vi "vy_animated_generater.vi"(4 "new attribute":T1(ring)=enum."grey", 5 "chage_leave":i32=-1, 6 "leaves":T3={"names"=["Cube", "Pyramid", "Sphere"], "shapes"=[[{"xyzd"=[1.0, 1.0, 1.0, 1.0], "attribute"=enum."red", "prev. Ind."=[0, 0]}, {"xyzd"=[-1.0, 1.0, 1.0, 1.0], "attribute"=enum."red", "prev. Ind."=[0, 0]}, {"xyzd"=[1.0, -1.0, 1.0, 1.0], "attribute"=enum."pink", "prev. Ind."=[-1, -2]}, {"xyzd"=[-1.0, -1.0, 1.0, 1.0], "attribute"=enum."pink", "prev. Ind."=[-2, -1]}, {"xyzd"=[-1.0, -1.0, -1.0, 1.0], "attribute"=enum."red", "prev. Ind."=[-3, -1]}, {"xyzd"=[-1.0, 1.0, -1.0, 1.0], "attribute"=enum."red", "prev. Ind."=[-4, -1]}, {"xyzd"=[1.0, -1.0, -1.0, 1.0], "attribute"=enum."red", "prev. Ind."=[-4, -6]}, {"xyzd"=[1.0, 1.0, -1.0, 1.0], "attribute"=enum."red", "prev. Ind."=[-1, -7]}, {"xyzd"=[-1.0, 1.0, -1.0, 1.0], "attribute"=enum."blue", "prev. Ind."=[-2, -1]}, {"xyzd"=[-1.0, -1.0, -1.0, 1.0], "attribute"=enum."blue", "prev. Ind."=[-3, -1]}, {"xyzd"=[1.0, -1.0, 1.0, 1.0], "attribute"=enum."yellow", "prev. Ind."=[-4, -6]}, {"xyzd"=[1.0, -1.0, 1.0, 1.0], "attribute"=enum."yellow", "prev. Ind."=[-2, -8]}, {"xyzd"=[1.0, 1.0, -1.0, 1.0], "attribute"=enum."green", "prev. Ind."=[-11, -4]}, {"xyzd"=[1.0, 1.0, -1.0, 1.0], "attribute"=enum."green", "prev. Ind."=[-13, -12]}, {"xyzd"=[], "attribute"=enum."none", "prev. Ind."=[]}, {"xyzd"=[], "attribute"=enum."none", "prev. Ind."=[]}, {"xyzd"=[], "attribute"=enum."none", "prev. Ind."=[]}, {"xyzd"=[], "attribute"=enum."none", "prev. Ind."=[]}, {"xyzd"=[], "attribute"=enum."none", "prev. Ind."=[]}, {"xyzd"=[], "attribute"=enum."none", "prev. Ind."=[]}, {"xyzd"=[], "attribute"=enum."none", "prev. Ind."=[]}, {"xyzd"=[], "attribute"=enum."none", "prev. Ind."=[]}, {"xyzd"=[], "attribute"=enum."none", "prev. Ind."=[]}, {"xyzd"=[], "attribute"=enum."none", "prev. Ind."=[]}, {"xyzd"=[], "attribute"=enum."none", "prev. Ind."=[]}, {"xyzd"=[], "attribute"=enum."none", "prev. Ind."=[]}, {"xyzd"=[], "attribute"=enum."none", "prev. Ind."=[]}, {"xyzd"=[], "attribute"=enum."none", "prev. Ind."=[]}, {"xyzd"=[], "attribute"=enum."none", "prev. Ind."=[]}, {"xyzd"=[], "attribute"=enum."none", "prev. Ind."=[]}, {"xyzd"=[], "attribute"=enum."none", "prev. Ind."=[]}, {"xyzd"=[], "attribute"=enum."none", "prev. Ind."=[]}, {"xyzd"=[], "attribute"=enum."none", "prev. Ind."=[]}, {"xyzd"=[], "attribute"=enum."none", "prev. Ind."=[]}, {"xyzd"=[], "attribute"=enum."none", "prev. Ind."=[]}, {"xyzd"=[], "attribute"=enum."none", "prev. Ind."=[]}, {"xyzd"=[], "attribute"=enum."none", "prev. Ind."=[]}, {"xyzd"=[], "attribute"=enum."none", "prev. Ind."=[]}, {"xyzd"=[], "attribute"=enum."none", "prev. Ind."=[]}, {"xyzd"=[], "attribute"=enum."none", "prev. Ind."=[]}, {"xyzd"=[], "attribute"=enum."none", "prev. Ind."=[]}, {"xyzd"=[], "attribute"=enum."none", "prev. Ind."=[]}, {"xyzd"=[], "attribute"=enum."none", "prev. Ind."=[]}, {"xyzd"=[], "attribute"=enum."none", "prev. Ind."=[]}, {"xyzd"=[], "attribute"=enum."none", "prev. Ind."=[]}, {"xyzd"=[], "attribute"=enum."none", "prev. Ind."=[]}, {"xyzd"=[], "attribute"=enum."none", "prev. Ind."=[]}, {"xyzd"=[], "attribute"=enum."none", "prev. Ind."=[]}, {"xyzd"=[], "attribute"=enum."none", "prev. Ind."=[]}, {"xyzd"=[], "attribute"=enum."none", "prev. Ind."=[]}, {"xyzd"=[], "attribute"=enum."none", "prev. Ind."=[]}, {"xyzd"=[], "attribute"=enum."none", "prev. Ind."=[]}, {"xyzd"=[], "attribute"=enum."none", "prev. Ind."=[]}, {"xyzd"=[], "attribute"=enum."none", "prev. Ind."=[]}, {"xyzd"=[], "attribute"=enum."none", "prev. Ind."=[]}, {"xyzd"=[], "attribute"=enum."none", "prev. Ind."=[]}, {"xyzd"=[], "attribute"=enum."none", "prev. Ind."=[]}, {"xyzd"=[], "attribute"=enum."none", "prev. Ind."=[]}, {"xyzd"=[], "attribute"=enum."none", "prev. Ind."=[]}, {"xyzd"=[], "attribute"=enum."none", "prev. Ind."=[]}, {"xyzd"=[], "attribute"=enum."none", "prev. Ind."=[]}, {"xyzd"=[], "attribute"=enum."none", "prev. Ind."=[]}, {"xyzd"=[], "attribute"=enum."none", "prev. Ind."=[]}, {"xyzd"=[], "attribute"=enum."none", "prev. Ind."=[]}, {"xyzd"=[], "attribute"=enum."none", "prev. Ind."=[]}, {"xyzd"=[], "attribute"=enum."none", "prev. Ind."=[]}, {"xyzd"=[], "attribute"=enum."none", "prev. Ind."=[]}, {"xyzd"=[], "attribute"=enum."none", "prev. Ind."=[]}, {"xyzd"=[], "attribute"=enum."none", "prev. Ind."=[]}, {"xyzd"=[], "attribute"=enum."none", "prev. Ind."=[]}, {"xyzd"=[], "attribute"=enum."none", "prev. Ind."=[]}, {"xyzd"=[], "attribute"=enum."none", "prev. Ind."=[]}, {"xyzd"=[], "attribute"=enum."none", "prev. Ind."=[]}, {"xyzd"=[], "attribute"=enum."none", "prev. Ind."=[]}, {"xyzd"=[], "attribute"=enum."none", "prev. Ind."=[]}, {"xyzd"=[], "attribute"=enum."none", "prev. Ind."=[]}, {"xyzd"=[], "attribute"=enum."none", "prev. Ind."=[]}, {"xyzd"=[], "attribute"=enum."none", "prev. Ind."=[]}, {"xyzd"=[], "attribute"=enum."none", "prev. Ind."=[]}, {"xyzd"=[], "attribute"=enum."none", "prev. Ind."=[]}], [{"xyzd"=[1.0, 1.0, 1.0, 1.0], "attribute"=enum."red", "prev. Ind."=[0, 0]}, {"xyzd"=[-1.0, 1.0, 1.0, 1.0], "attribute"=enum."red", "prev. Ind."=[0, 0]}, {"xyzd"=[1.0, -1.0, 1.0, 1.0], "attribute"=enum."red", "prev. Ind."=[-1, -2]}, {"xyzd"=[-1.0, -1.0, 1.0, 1.0], "attribute"=enum."red", "prev. Ind."=[-2, -1]}, {"xyzd"=[0.0, 0.0, -1.0, 1.0], "attribute"=enum."yellow", "prev. Ind."=[-4, -3]}, {"xyzd"=[0.0, 0.0, -1.0, 1.0], "attribute"=enum."red", "prev. Ind."=[-3, -5]}, {"xyzd"=[0.0, 0.0, -1.0, 1.0], "attribute"=enum."yellow", "prev. Ind."=[-3, -4]}, {"xyzd"=[0.0, 0.0, -1.0, 1.0], "attribute"=enum."red", "prev. Ind."=[-6, -4]}, {"xyzd"=[], "attribute"=enum."none", "prev. Ind."=[]}, {"xyzd"=[], "attribute"=enum."none", "prev. Ind."=[]}, {"xyzd"=[], "attribute"=enum."none", "prev. Ind."=[]}, {"xyzd"=[], "attribute"=enum."none", "prev. Ind."=[]}, {"xyzd"=[], "attribute"=enum."none", "prev. Ind."=[]}, {"xyzd"=[], "attribute"=enum."none", "prev. Ind."=[]}, {"xyzd"=[], "attribute"=enum."none", "prev. Ind."=[]}, {"xyzd"=[], "attribute"=enum."none", "prev. Ind."=[]}, {"xyzd"=[], "attribute"=enum."none", "prev. Ind."=[]}, {"xyzd"=[], "attribute"=enum."none", "prev. Ind."=[]}, {"xyzd"=[], "attribute"=enum."none", "prev. Ind."=[]}, {"xyzd"=[], "attribute"=enum."none", "prev. Ind."=[]}, {"xyzd"=[], "attribute"=enum."none", "prev. Ind."=[]}, {"xyzd"=[], "attribute"=enum."none", "prev. Ind."=[]}, {"xyzd"=[], "attribute"=enum."none", "prev. Ind."=[]}, {"xyzd"=[], "attribute"=enum."none", "prev. Ind."=[]}, {"xyzd"=[], "attribute"=enum."none", "prev. Ind."=[]}, {"xyzd"=[], "attribute"=enum."none", "prev. Ind."=[]}, {"xyzd"=[], "attribute"=enum."none", "prev. Ind."=[]}, {"xyzd"=[], "attribute"=enum."none", "prev. Ind."=[]}, {"xyzd"=[], "attribute"=enum."none", "prev. Ind."=[]}, {"xyzd"=[], "attribute"=enum."none", "prev. Ind."=[]}, {"xyzd"=[], "attribute"=enum."none", "prev. Ind."=[]}, {"xyzd"=[], "attribute"=enum."none", "prev. Ind."=[]}, {"xyzd"=[], "attribute"=enum."none", "prev. Ind."=[]}, {"xyzd"=[], "attribute"=enum."none", "prev. Ind."=[]}, {"xyzd"=[], "attribute"=enum."none", "prev. Ind."=[]}, {"xyzd"=[], "attribute"=enum."none", "prev. Ind."=[]}, {"xyzd"=[], "attribute"=enum."none", "prev. Ind."=[]}, {"xyzd"=[], "attribute"=enum."none", "prev. Ind."=[]}, {"xyzd"=[], "attribute"=enum."none", "prev. Ind."=[]}, {"xyzd"=[], "attribute"=enum."none", "prev. Ind."=[]}, {"xyzd"=[], "attribute"=enum."none", "prev. Ind."=[]}, {"xyzd"=[], "attribute"=enum."none", "prev. Ind."=[]}, {"xyzd"=[], "attribute"=enum."none", "prev. Ind."=[]}, {"xyzd"=[], "attribute"=enum."none", "prev. Ind."=[]}, {"xyzd"=[], "attribute"=enum."none", "prev. Ind."=[]}, {"xyzd"=[], "attribute"=enum."none", "prev. Ind."=[]}, {"xyzd"=[], "attribute"=enum."none", "prev. Ind."=[]}, {"xyzd"=[], "attribute"=enum."none", "prev. Ind."=[]}, {"xyzd"=[], "attribute"=enum."none", "prev. Ind."=[]}, {"xyzd"=[], "attribute"=enum."none", "prev. Ind."=[]}, {"xyzd"=[], "attribute"=enum."none", "prev. Ind."=[]}, {"xyzd"=[], "attribute"=enum."none", "prev. Ind."=[]}, {"xyzd"=[], "attribute"=enum."none", "prev. Ind."=[]}, {"xyzd"=[], "attribute"=enum."none", "prev. Ind."=[]}, {"xyzd"=[], "attribute"=enum."none", "prev. Ind."=[]}, {"xyzd"=[], "attribute"=enum."none", "prev. Ind."=[]}, {"xyzd"=[], "attribute"=enum."none", "prev. Ind."=[]}, {"xyzd"=[], "attribute"=enum."none", "prev. Ind."=[]}, {"xyzd"=[], "attribute"=enum."none", "prev. Ind."=[]}, {"xyzd"=[], "attribute"=enum."none", "prev. Ind."=[]}, {"xyzd"=[], "attribute"=enum."none", "prev. Ind."=[]}, {"xyzd"=[], "attribute"=enum."none", "prev. Ind."=[]}, {"xyzd"=[], "attribute"=enum."none", "prev. Ind."=[]}, {"xyzd"=[], "attribute"=enum."none", "prev. Ind."=[]}, {"xyzd"=[], "attribute"=enum."none", "prev. Ind."=[]}, {"xyzd"=[], "attribute"=enum."none", "prev. Ind."=[]}, {"xyzd"=[], "attribute"=enum."none", "prev. Ind."=[]}, {"xyzd"=[], "attribute"=enum."none", "prev. Ind."=[]}, {"xyzd"=[], "attribute"=enum."none", "prev. Ind."=[]}, {"xyzd"=[], "attribute"=enum."none", "prev. Ind."=[]}, {"xyzd"=[], "attribute"=enum."none", "prev. Ind."=[]}, {"xyzd"=[], "attribute"=enum."none", "prev. Ind."=[]}, {"xyzd"=[], "attribute"=enum."none", "prev. Ind."=[]}, {"xyzd"=[], "attribute"=enum."none", "prev. Ind."=[]}, {"xyzd"=[], "attribute"=enum."none", "prev. Ind."=[]}, {"xyzd"=[], "attribute"=enum."none", "prev. Ind."=[]}, {"xyzd"=[], "attribute"=enum."none", "prev. Ind."=[]}, {"xyzd"=[], "attribute"=enum."none", "prev. Ind."=[]}, {"xyzd"=[], "attribute"=enum."none", "prev. Ind."=[]}, {"xyzd"=[], "attribute"=enum."none", "prev. Ind."=[]}], [{"xyzd"=[-0.09090909090909091, 0.0, -1.0, 1.0], "attribute"=enum."red", "prev. Ind."=[0, 0]}, {"xyzd"=[0.09090909090909091, 0.0, -1.0, 1.0], "attribute"=enum."red", "prev. Ind."=[0, 0]}, {"xyzd"=[0.0, 0.09090909090909091, -1.0, 1.0], "attribute"=enum."red", "prev. Ind."=[-1, -2]}, {"xyzd"=[1.1132785034748885e-17, -0.09090909090909091, -1.0, 1.0], "attribute"=enum."red", "prev. Ind."=[-2, -3]}, {"xyzd"=[0.22076356771783573, 0.2162289295654466, -0.9510565162951535, 1.0], "attribute"=enum."red", "prev. Ind."=[-2, -3]}, {"xyzd"=[0.2162289295654466, -0.2207635677178357, -0.9510565162951535, 1.0], "attribute"=enum."red", "prev. Ind."=[-4, -2]}, {"xyzd"=[-0.2207635677178357, -0.21622892956544665, -0.9510565162951535, 1.0], "attribute"=enum."red", "prev. Ind."=[-3, -6]}, {"xyzd"=[-0.21622892956544673, 0.2207635677178356, -0.9510565162951535, 1.0], "attribute"=enum."red", "prev. Ind."=[-7, -5]}, {"xyzd"=[0.3494270285103859, 0.4726438982563176, -0.8090169943749475, 1.0], "attribute"=enum."red", "prev. Ind."=[-6, -4]}, {"xyzd"=[0.5873920684232319, 0.021495598758897283, -0.8090169943749475, 1.0], "attribute"=enum."red", "prev. Ind."=[-4, -5]}, {"xyzd"=[0.3830389001987991, -0.44583932503427814, -0.8090169943749475, 1.0], "attribute"=enum."red", "prev. Ind."=[-1, -5]}, {"xyzd"=[-0.10975037244495894, -0.5774481436118044, -0.8090169943749475, 1.0], "attribute"=enum."red", "prev. Ind."=[-6, -5]}, {"xyzd"=[-0.5198953761380584, -0.274226732254157, -0.8090169943749475, 1.0], "attribute"=enum."red", "prev. Ind."=[-1, -6]}, {"xyzd"=[-0.5385485576662208, 0.23549300169677978, -0.8090169943749475, 1.0], "attribute"=enum."red", "prev. Ind."=[-1, -6]}, {"xyzd"=[-0.1516636908831792, 0.5678817021882443, -0.8090169943749475, 1.0], "attribute"=enum."red", "prev. Ind."=[-1, -7]}, {"xyzd"=[0.6603788169001088, 0.467341754369419, -0.5877852522924731, 1.0], "attribute"=enum."red", "prev. Ind."=[-6, -7]}, {"xyzd"=[0.806281012237646, -0.06647876723067801, -0.5877852522924731, 1.0], "attribute"=enum."red", "prev. Ind."=[-1, -7]}, {"xyzd"=[0.5749153611338783, -0.5691931348143405, -0.5877852522924731, 1.0], "attribute"=enum."red", "prev. Ind."=[-1, -7]}, {"xyzd"=[0.07454042308304981, -0.805575708741316, -0.5877852522924731, 1.0], "attribute"=enum."red", "prev. Ind."=[-8, -7]}, {"xyzd"=[-0.46071280735286246, -0.6650204555714944, -0.5877852522924731, 1.0], "attribute"=enum."red", "prev. Ind."=[-7, -8]}, {"xyzd"=[-0.7803933949758588, -0.2132947403606729, -0.5877852522924731, 1.0], "attribute"=enum."red", "prev. Ind."=[-1, -8]}, {"xyzd"=[-0.7349192399831584, 0.33823395437189707, -0.5877852522924731, 1.0], "attribute"=enum."red", "prev. Ind."=[-1, -8]}, {"xyzd"=[-0.34556820488478407, 0.7314992228021719, -0.5877852522924731, 1.0], "attribute"=enum."red", "prev. Ind."=[-1, -8]}, {"xyzd"=[0.20547803384198088, 0.7824878751750135, -0.5877852522924731, 1.0], "attribute"=enum."red", "prev. Ind."=[-9, -15]}, {"xyzd"=[0.43703805980741456, 0.8446929805954613, -0.3090169943749474, 1.0], "attribute"=enum."red", "prev. Ind."=[-9, -1]}, {"xyzd"=[0.8243353153228079, 0.4743203401701433, -0.3090169943749474, 1.0], "attribute"=enum."red", "prev. Ind."=[-1, -10]}, {"xyzd"=[0.9499119326982213, -0.0466456568718201, -0.3090169943749474, 1.0], "attribute"=enum."red", "prev. Ind."=[-1, -10]}, {"xyzd"=[0.77389822319894, -0.5528019874394424, -0.3090169943749474, 1.0], "attribute"=enum."red", "prev. Ind."=[-1, -10]}, {"xyzd"=[0.3521772959375426, -0.8834475929072387, -0.3090169943749474, 1.0], "attribute"=enum."red", "prev. Ind."=[-11, -10]}, {"xyzd"=[-0.18135743441815916, -0.9336048297693927, -0.3090169943749474, 1.0], "attribute"=enum."red", "prev. Ind."=[-10, -11]}, {"xyzd"=[-0.657312460756494, -0.6873491297162718, -0.3090169943749474, 1.0], "attribute"=enum."red", "prev. Ind."=[-1, -11]}, {"xyzd"=[-0.9245754251525565, -0.22286493755510975, -0.3090169943749474, 1.0], "attribute"=enum."red", "prev. Ind."=[-1, -11]}, {"xyzd"=[-0.8982922248004648, 0.3123772975913979, -0.3090169943749474, 1.0], "attribute"=enum."red", "prev. Ind."=[-1, -11]}, {"xyzd"=[-0.5868075901037884, 0.7484419479051518, -0.3090169943749474, 1.0], "attribute"=enum."red", "prev. Ind."=[-12, -11]}, {"xyzd"=[-0.0890156917334638, 0.9468815679971211, -0.3090169943749474, 1.0], "attribute"=enum."red", "prev. Ind."=[-11, -12]}, {"xyzd"=[0.0, 1.0, 0.0, 1.0], "attribute"=enum."red", "prev. Ind."=[-11, -1]}, {"xyzd"=[0.49999999999999994, 0.8660254037844387, 0.0, 1.0], "attribute"=enum."red", "prev. Ind."=[-1, -12]}, {"xyzd"=[0.8660254037844386, 0.5000000000000001, 0.0, 1.0], "attribute"=enum."red", "prev. Ind."=[-1, -12]}, {"xyzd"=[1.0, 6.123031769111886e-17, 0.0, 1.0], "attribute"=enum."red", "prev. Ind."=[-1, -12]}, {"xyzd"=[0.8660254037844387, -0.4999999999999998, 0.0, 1.0], "attribute"=enum."red", "prev. Ind."=[-1, -12]}, {"xyzd"=[0.49999999999999994, -0.8660254037844387, 0.0, 1.0], "attribute"=enum."red", "prev. Ind."=[-1, -12]}, {"xyzd"=[1.2246063538223773e-16, -1.0, 0.0, 1.0], "attribute"=enum."red", "prev. Ind."=[-13, -12]}, {"xyzd"=[-0.5000000000000001, -0.8660254037844386, 0.0, 1.0], "attribute"=enum."red", "prev. Ind."=[-13, -12]}, {"xyzd"=[-0.8660254037844384, -0.5000000000000004, 0.0, 1.0], "attribute"=enum."red", "prev. Ind."=[-12, -13]}, {"xyzd"=[-1.0, -1.836909530733566e-16, 0.0, 1.0], "attribute"=enum."red", "prev. Ind."=[-12, -13]}, {"xyzd"=[-0.8660254037844386, 0.5000000000000001, 0.0, 1.0], "attribute"=enum."red", "prev. Ind."=[-12, -13]}, {"xyzd"=[-0.5000000000000004, 0.8660254037844384, 0.0, 1.0], "attribute"=enum."red", "prev. Ind."=[-1, -13]}, {"xyzd"=[0.0, 0.9510565162951535, 0.3090169943749474, 1.0], "attribute"=enum."red", "prev. Ind."=[-11, -12]}, {"xyzd"=[0.5141799724162847, 0.8000796542554137, 0.3090169943749474, 1.0], "attribute"=enum."red", "prev. Ind."=[-1, -12]}, {"xyzd"=[0.8651114366124775, 0.39508315508228004, 0.3090169943749474, 1.0], "attribute"=enum."red", "prev. Ind."=[-11, -12]}, {"xyzd"=[0.9413761322695258, -0.13534945430529863, 0.3090169943749474, 1.0], "attribute"=enum."red", "prev. Ind."=[-11, -12]}, {"xyzd"=[0.718760557376906, -0.6228095682844902, 0.3090169943749474, 1.0], "attribute"=enum."red", "prev. Ind."=[-11, -12]}, {"xyzd"=[0.2679435840365368, -0.9125320448954815, 0.3090169943749474, 1.0], "attribute"=enum."red", "prev. Ind."=[-11, -12]}, {"xyzd"=[-0.2679435840365362, -0.9125320448954817, 0.3090169943749474, 1.0], "attribute"=enum."red", "prev. Ind."=[-12, -11]}, {"xyzd"=[-0.7187605573769059, -0.6228095682844903, 0.3090169943749474, 1.0], "attribute"=enum."red", "prev. Ind."=[-12, -11]}, {"xyzd"=[-0.9413761322695257, -0.13534945430529882, 0.3090169943749474, 1.0], "attribute"=enum."red", "prev. Ind."=[-12, -11]}, {"xyzd"=[-0.8651114366124774, 0.39508315508228037, 0.3090169943749474, 1.0], "attribute"=enum."red", "prev. Ind."=[-12, -11]}, {"xyzd"=[-0.5141799724162853, 0.8000796542554134, 0.3090169943749474, 1.0], "attribute"=enum."red", "prev. Ind."=[-1, -11]}, {"xyzd"=[0.0, 0.8090169943749475, 0.5877852522924731, 1.0], "attribute"=enum."red", "prev. Ind."=[-10, -11]}, {"xyzd"=[0.5200261000100609, 0.619742972929746, 0.5877852522924731, 1.0], "attribute"=enum."red", "prev. Ind."=[-10, -11]}, {"xyzd"=[0.7967262083790821, 0.14048432677478692, 0.5877852522924731, 1.0], "attribute"=enum."none", "prev. Ind."=[-10, -11]}, {"xyzd"=[0.7006292692220368, -0.40450849718747356, 0.5877852522924731, 1.0], "attribute"=enum."none", "prev. Ind."=[-11, -10]}, {"xyzd"=[0.27670010836902137, -0.7602272997045328, 0.5877852522924731, 1.0], "attribute"=enum."none", "prev. Ind."=[-11, -10]}, {"xyzd"=[-0.2767001083690212, -0.760227299704533, 0.5877852522924731, 1.0], "attribute"=enum."none", "prev. Ind."=[-9, -10]}, {"xyzd"=[-0.7006292692220366, -0.40450849718747406, 0.5877852522924731, 1.0], "attribute"=enum."none", "prev. Ind."=[-9, -10]}, {"xyzd"=[-0.7967262083790823, 0.14048432677478656, 0.5877852522924731, 1.0], "attribute"=enum."red", "prev. Ind."=[-10, -9]}, {"xyzd"=[-0.5200261000100611, 0.6197429729297458, 0.5877852522924731, 1.0], "attribute"=enum."red", "prev. Ind."=[-10, -9]}, {"xyzd"=[0.0, 0.5877852522924731, 0.8090169943749475, 1.0], "attribute"=enum."red", "prev. Ind."=[-8, -9]}, {"xyzd"=[0.45954901517266916, 0.3664781104873198, 0.8090169943749475, 1.0], "attribute"=enum."red", "prev. Ind."=[-8, -9]}, {"xyzd"=[0.5730482488287673, -0.13079452330586896, 0.8090169943749475, 1.0], "attribute"=enum."red", "prev. Ind."=[-9, -8]}, {"xyzd"=[0.25503046306281557, -0.5295762133276872, 0.8090169943749475, 1.0], "attribute"=enum."red", "prev. Ind."=[-1, -8]}, {"xyzd"=[-0.2550304630628154, -0.5295762133276873, 0.8090169943749475, 1.0], "attribute"=enum."red", "prev. Ind."=[-1, -8]}, {"xyzd"=[-0.5730482488287673, -0.13079452330586913, 0.8090169943749475, 1.0], "attribute"=enum."red", "prev. Ind."=[-7, -8]}, {"xyzd"=[-0.4595490151726693, 0.3664781104873197, 0.8090169943749475, 1.0], "attribute"=enum."red", "prev. Ind."=[-8, -7]}, {"xyzd"=[0.0, 0.30901699437494745, 0.9510565162951535, 1.0], "attribute"=enum."red", "prev. Ind."=[-6, -7]}, {"xyzd"=[0.30901699437494745, 1.8921208737532724e-17, 0.9510565162951535, 1.0], "attribute"=enum."red", "prev. Ind."=[-7, -6]}, {"xyzd"=[3.784241747506545e-17, -0.30901699437494745, 0.9510565162951535, 1.0], "attribute"=enum."red", "prev. Ind."=[-5, -6]}, {"xyzd"=[-0.30901699437494745, -5.676362621259817e-17, 0.9510565162951535, 1.0], "attribute"=enum."red", "prev. Ind."=[-4, -5]}, {"xyzd"=[0.0, 0.09090909090909091, 1.0, 1.0], "attribute"=enum."red", "prev. Ind."=[-3, -4]}, {"xyzd"=[1.1132785034748885e-17, -0.09090909090909091, 1.0, 1.0], "attribute"=enum."red", "prev. Ind."=[-3, -1]}]]}, 7 "variables":dbl[](array[numeric])=[0.4925750394941765, 0.002174868167709741, 0.5074249605058234], 8 "vy_string":string="Structure  { s=(15,15,15)} [klossar {m=(,v1*3,) r=(30,v0*360,0)}  [Pyramid{r=(,,v0*360) m=(,,-4)} Cube {s=(1,v1,1) m=(,2-v1,)} Pyramid{r=(,180,v0*360) m=(,,4)}]  Cube{r=(45,v1*90,) m=(v1*5-2,-5,)}]", 9 "vy_in":T2(array[cluster])) -> (0 "selected leave":string, 3 "vy_out":T2(array[cluster]))   [LabVIEW 2011]
uses:
  <vilib>/Analysis/baseanly.llb/A x Vector.vi
  <vilib>/Analysis/NI_AALBase.lvlib
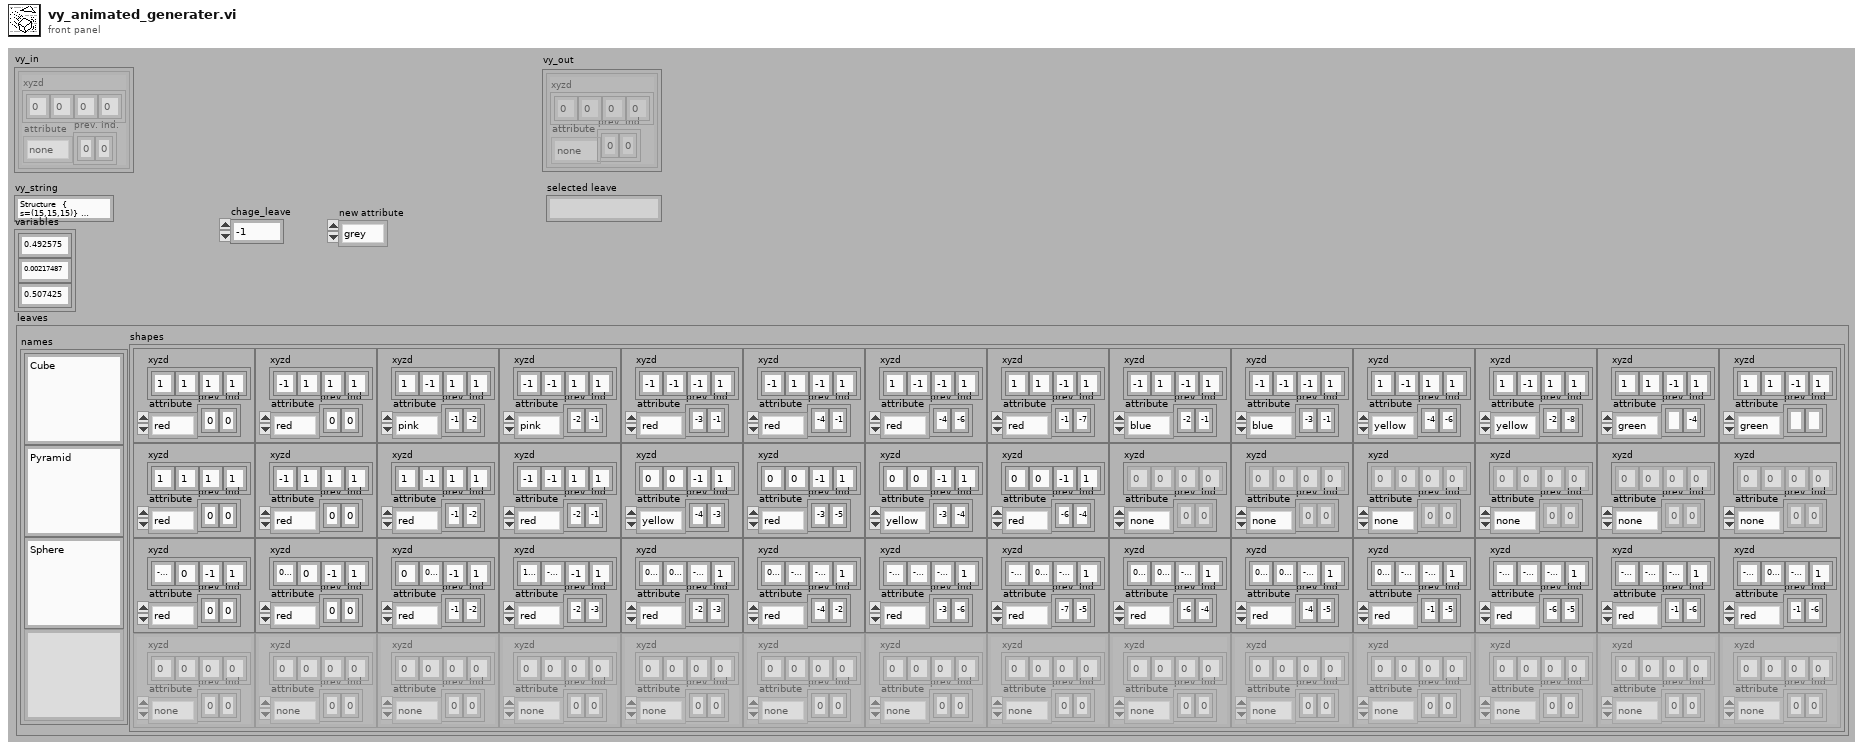
[diagram p1: front panel]
types:
  T1 = enum16{"none", "transparent", "reflective", "white", "black", "grey", "red", "yellow", "green", "blue", "pink"}
  T2 = cluster{"xyzd":dbl[], "attribute":enum16{"none", "transparent", "reflective", "white", "black", "grey", "red", "yellow", "green", "blue", "pink"}, "prev. Ind.":i16[]}[]
  T3 = cluster{"names":string[], "shapes":cluster{"xyzd":dbl[], "attribute":enum16{"none", "transparent", "reflective", "white", "black", "grey", "red", "yellow", "green", "blue", "pink"}, "prev. Ind.":i16[]}[][]}
  T4 = cluster{"xyzd":dbl[], "attribute":enum16{"none", "transparent", "reflective", "white", "black", "grey", "red", "yellow", "green", "blue", "pink"}, "prev. Ind.":i16[]}[][]
  T5 = cluster{"xyzd":dbl[], "attribute":enum16{"none", "transparent", "reflective", "white", "black", "grey", "red", "yellow", "green", "blue", "pink"}, "prev. Ind.":i16[]}
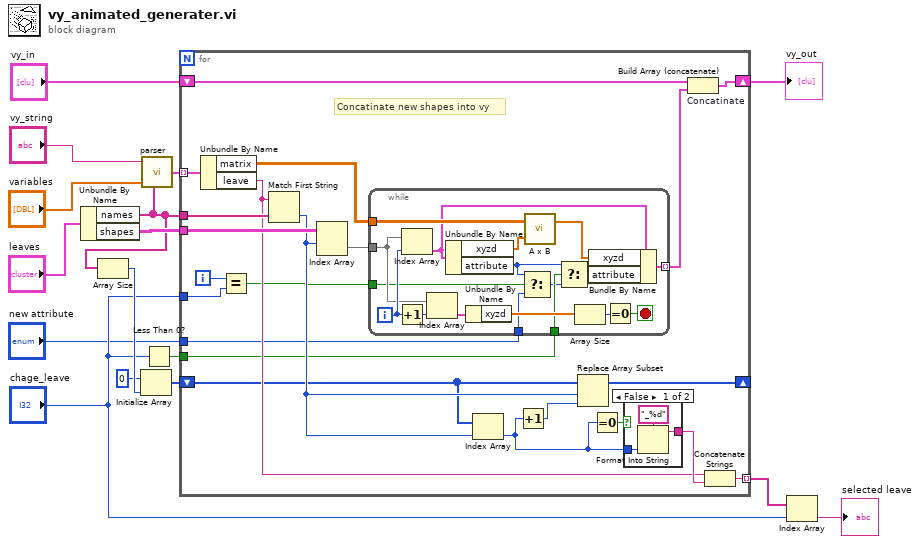
[diagram p0: block diagram]
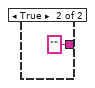
[diagram p2: hidden frame]
diagram:
  n1 = Unbundle By Name("leaves") -> ("names"=w12:string[], "shapes"=w14:T4)
  n2 = Array Size(array=w12) -> (size(s)=w11:i32)
  n3 = Initialize Array(0, w11) -> (w9:i32[])
  n4 = call "parser.vi"("in string"="vy_string", "variables"="variables", "leaves"=w12) -> ("leaves_projection_array"=w13:cluster{"matrix":dbl[][], "leave":string}[])  [unwired: 2 in]
  n5 = Less Than 0?(x="chage_leave") -> (x < 0?=w2:bool)
  n6 = for {
    tunnel: w13 -> [w38] mode=indexing
    tunnel: w12 -> [w37]
    tunnel: w14 -> [w36]
    shift-right: [w33] -> w6
    shift-left: "vy_in" -> [w32]
    tunnel: [w29] -> w5 mode=indexing
    shift-right: [w24] -> _
    shift-left: w9 -> [w25]
    tunnel: "chage_leave" -> [w20]
    tunnel: "new attribute" -> [w17]
    tunnel: w2 -> [w18]
    i -> [w21]
    # "Concatinate new shapes into vy"
    n7 = Unbundle By Name(w38) -> ("matrix"=w34:dbl[][], "leave"=w28:string)
    n8 = Equal?(x=w21, y=w20) -> (x = y?=w19:bool)
    n9 = Match First String(2:w37, 3:w28) -> (0:w26:i32)  [unwired: 1 out]
    n10 = Index Array(array=w36, index (row)=w26) -> (element=w35:T2)  [unwired: 1 in]
    n11 = while {
      tunnel: w35 -> [w51]
      tunnel: w34 -> [w60]
      tunnel: [w58] -> w31 mode=indexing
      tunnel: w17 -> [w48]
      tunnel: w19 -> [w47]
      tunnel: w18 -> [w46]
      i -> [w53]
      stop <- w54 stop-if-true
      n12 = Increment(x=w53) -> (x+1=w52:i32)
      n13 = Index Array(array=w51, index=w53) -> (element=w57:T5)
      n14 = Index Array(array=w51, index=w52) -> (element=w50:T5)
      n15 = Unbundle By Name(w57) -> ("xyzd"=w56:dbl[], "attribute"=w43:T1)
      n16 = Unbundle By Name(w50) -> ("xyzd"=w49:dbl[])
      n17 = Select(t=w43, s=w47, f=w48) -> (s? t:f=w44:T1)
      n18 = call-poly <vilib>:"A x B.vi"("Vector"=w56, "A"=w60) -> ("A x Vector"=w59:dbl[])  [unwired: 1 out]
      n19 = Select(t=w43, s=w46, f=w44) -> (s? t:f=w45:T1)
      n20 = Array Size(array=w49) -> (size(s)=w55:i32)
      n21 = Bundle By Name(cluster=w57, "xyzd"=w59, "attribute"=w45) -> (w58:T5)
      n22 = Equal To 0?(x=w55) -> (x = 0?=w54:bool)
    }
    n23 = Index Array(array=w25, index=w26) -> (element=w23:i32)
    n24 = Increment(x=w23) -> (x+1=w27:i32)
    n25 = Replace Array Subset(array=w25, new element=w27, index=w26) -> (w24:i32[])
    n26 = Equal To 0?(x=w23) -> (x = 0?=w22:bool)
    n27 = case shown="False" w22 {
      tunnel: [w40 ""] -> w30
      tunnel: w23 -> [w39 _]
      frame False {
        n28 = Format Into String(format string="_%d", w39) -> (resulting string=w40:string)  [unwired: 2 in, 1 out]
      }
      frame True {
      }
    }
    n29 = Build Array (concatenate) "Concatinate"(w32, w31) -> (w33:T2)
    n30 = Concatenate Strings(w28, w30) -> (w29:string)
  }
  "vy_out" <- w6
  n31 = Index Array(array=w5, index="chage_leave") -> (element=→"selected leave":string)
